vi "Read session reservation in.vi"(0 "AbstractDMM in":refnum<class "AbstractDMM.lvclass">, 11 "error in (no error)":errorcluster) -> (4 "AbstractDMM out":refnum<class "AbstractDMM.lvclass">, 6 "MeasurementLink Session Management V1.lvlib:Session Reservation.lvclass":refnum<class "Session Reservation.lvclass">, 15 "error out":errorcluster)   [LabVIEW 2020, in "AbstractDMM.lvlib" / "AbstractDMM.lvclass"]
uses:
  AbstractDMM.lvclass
  <vilib>/MeasurementLink/MeasurementLink Session Management V1/Session Reservation/Session Reservation.lvclass
  AbstractDMM.lvclass/AbstractDMM.ctl
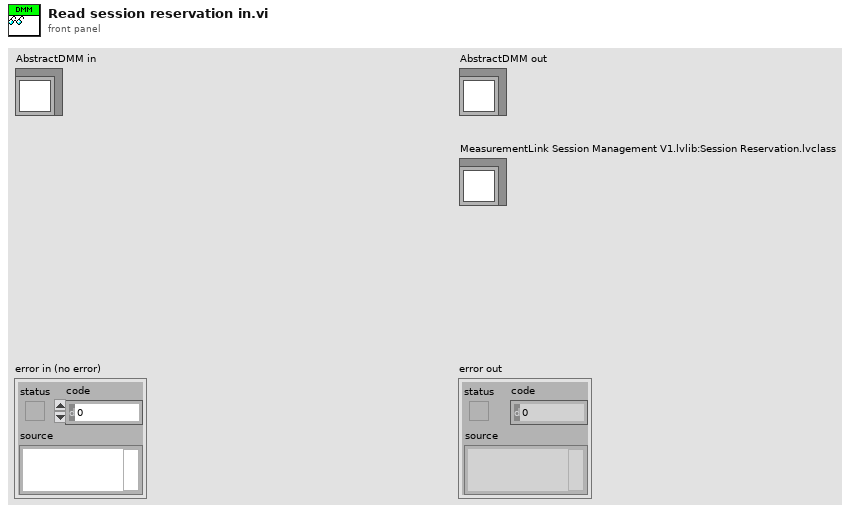
[diagram p1: front panel]
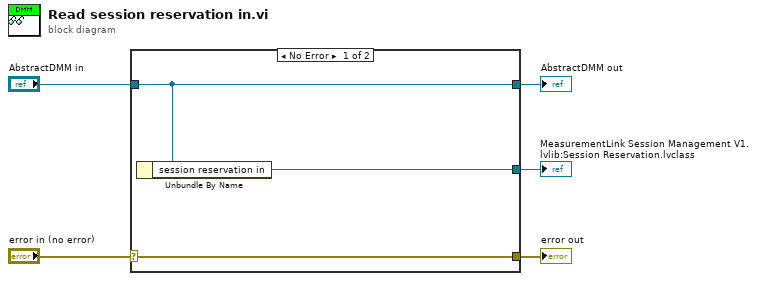
[diagram p0: block diagram]
diagram:
  n1 = case shown="No Error" "error in (no error)" {
    selector: "error in (no error)" -> [w8 w9]
    tunnel: [w8 w9] -> w4
    tunnel: [w7 w10] -> w2
    tunnel: "AbstractDMM in" -> [w7 w10]
    tunnel: [w6 _] -> w1
    frame No Error {
      n2 = Unbundle By Name(w7) -> ("session reservation in"=w6:refnum<class "Session Reservation.lvclass">)
    }
    frame Error {
    }
  }
  "error out" <- w4
  "AbstractDMM out" <- w2
  "MeasurementLink Session Management V1.lvlib:Session Reservation.lvclass" <- w1
